vi "Auto Align With Limelight.vi"(0 "Robot Velocities In":T1) -> (7 "Robot Velocities Out":T1, 8 "Rotational Velocity":dbl format="%.2f")   [LabVIEW 2020]
uses:
  Type Definitions/Data/Robot Velocities.ctl
  <vilib>/Rock Robotics/Network Tables/NT Read Number.vi
panel:
  out "Err/Out Chart":cluster{dbl, dbl}(graph)
  out "SP/PV Chart":cluster{"setpoint":dbl, "process variable":dbl}(graph)
  in  "PID gains":T2={"proportional gain (Kp)"=1.0, "integral time (Ki)"=0.0, "derivative time (Kd)"=0.0} {"derivative time (Kd)" format="%.3f"; "integral time (Ki)" format="%.3f"; "proportional gain (Kp)" format="%.3f"}
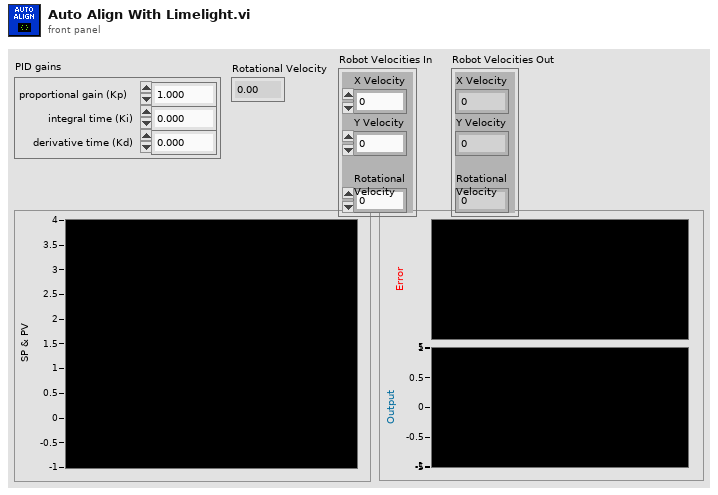
[diagram p1: front panel]
types:
  T1 = typedef "Robot Velocities.ctl" = cluster{"X Velocity":dbl, "Y Velocity":dbl, "Rotational \nVelocity":dbl}
  T2 = cluster{"proportional gain (Kp)":dbl, "integral time (Ki)":dbl, "derivative time (Kd)":dbl}
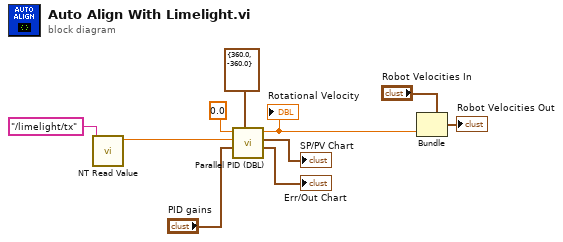
[diagram p0: block diagram]
diagram:
  n1 = call-poly <vilib>:"NT Read Value.vi"("name"="/limelight/tx" ("Name")) -> ("value"=w7:dbl)  [unwired: 8 in, 2 out]
  n2 = call <vilib>:"Parallel PID (DBL).vi"("output range"=cluster{"high":dbl, "low":dbl} {"high"=360.0, "low"=-360.0}, "PID gains"="PID gains", "process variable"=w7, "setpoint"=0.0) -> ("Err/Out Chart"=→"Err/Out Chart":cluster{dbl, dbl}, "SP/PV Chart"=→"SP/PV Chart":cluster{"setpoint":dbl, "process variable":dbl}, "output"=w2:dbl)  [unwired: 4 in, 1 out]
  "Rotational Velocity" <- w2
  n3 = Bundle(cluster="Robot Velocities In", "Rotational \nVelocity"=w2) -> (→"Robot Velocities Out":T1)  [unwired: 2 in]
